vi "Cleanup.vi"(0 "WaveformAddressSpace in":refnum<class "WaveformAddressSpace.lvclass">) -> (4 "WaveformAddressSpace out":refnum<class "WaveformAddressSpace.lvclass">)   [LabVIEW 2015, in "WaveformAddressSpace.lvclass"]
uses:
  WaveformAddressSpace.lvclass
  WaveformAddressSpace.lvclass/WaveformAddressSpace.ctl
  <vilib>/rvi/DataTransferAndStorage/Container/Common/niFpgaContainerExecOnDevCompGetState.vi
  <vilib>/rvi/Emulation/niFpgaEmulationIsFPGAContextNoSignature.vi
  <vilib>/rvi/DataTransferAndStorage/Container/Common/niFpgaContainerGetUniqueNameForEmu.vi
  <vilib>/rvi/Memory/Memory_Emulation/niFpgaMemoryEmulationCacheClearOnFirstRun.vi
  <vilib>/rvi/Memory/Memory_Emulation/nirvimemoryEmulationManagerCache_MakeExclusive.vi
  <vilib>/rvi/Memory/Memory_Emulation/niFpgaMemoryEmulationValidateCache.vi
  <vilib>/rvi/Memory/Memory_Emulation/nirvimemoryEmulationManagerCache_InsertValue.vi
  <vilib>/Utility/error.llb/Clear Errors.vi
  <vilib>/rvi/Memory/Memory_Emulation/nirvimemoryEmulationManagerCache_ReleaseExclusive.vi
  <vilib>/rvi/Memory/Memory_Emulation/nirvimemoryEmulationManagerCache_GetValue.vi
  <vilib>/rvi/Memory/Memory_Emulation/nirvimemoryEmulationManagerCache_SetValue.vi
  <vilib>/rvi/Emulation/niFpgaProcessEmulError.vi
  <vilib>/rvi/Emulation/niFpgaSctlEmulationGetInTimedLoop.vi
  <vilib>/rvi/DataTransferAndStorage/Container/XNode/niFpgaContainer.xnode
  <vilib>/rvi/DataTransferAndStorage/Register/Emulation/niFpgaRegisterEmulationRefIn.vi
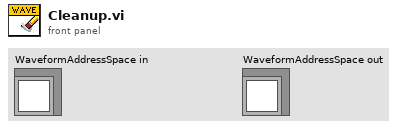
[diagram p1: front panel]
types:
  T1 = typedef "WaveformAddressSpace.lvclass/Registers.ctl" = cluster{"oclk_freq":refnum<k21>, "data_rate":refnum<k21>, "oclk_div":refnum<k21>, "oclk_mult":refnum<k21>, "AcquisitionType":refnum<k21>, "SamplesPerChan":refnum<k21>, "NumberOfChannels":refnum<k21>, "stop":refnum<k21>, "FIFO":refnum<k21>, "FirstRead":refnum<k21>, "ErrorCode":refnum<k21>, "ChannelCount":refnum<k21>, "Finished":refnum<k21>, "DMA_FIFO_Full":refnum<k21>, "ModuleUnderflow":refnum<k21>, "ConfigReadyIRQ":refnum<k21>, "ConfigReadyAck":refnum<k21>, "SynchStartIRQ":refnum<k21>, "SynchStartAck":refnum<k21>, "UnderflowCount":refnum<k21>, "FirstReadReset":refnum<k21>}
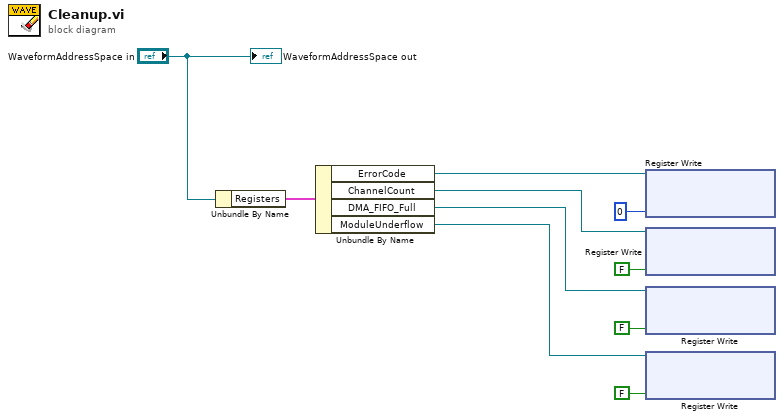
[diagram p0: block diagram]
diagram:
  n1 = Unbundle By Name("WaveformAddressSpace in") -> ("Registers"=w2:T1)
  n2 = Unbundle By Name(w2) -> ("ErrorCode"=w10:refnum<k21>, "ChannelCount"=w8:refnum<k21>, "DMA_FIFO_Full"=w6:refnum<k21>, "ModuleUnderflow"=w4:refnum<k21>)
  n3 = xnode ("Register Write")("Data"=0, "Register In"=w10) -> ()  [unwired: 1 out]
  n4 = xnode ("Register Write")("Data"=FALSE, "Register In"=w8) -> ()  [unwired: 1 out]
  n5 = xnode ("Register Write")("Data"=FALSE, "Register In"=w6) -> ()  [unwired: 1 out]
  n6 = xnode ("Register Write")("Data"=FALSE, "Register In"=w4) -> ()  [unwired: 1 out]
  "WaveformAddressSpace out" <- "WaveformAddressSpace in"
